vi "All Values.vi"(8 "error in (no error)":errorcluster, 11 "Group in":refnum<class "Group DBL.lvclass">) -> (0 "error out":errorcluster, 1 "Timestamp":dbl[](array[numeric]), 2 "Scaled":dbl[](array[numeric]), 3 "Group out":refnum<class "Group DBL.lvclass">, 4 "Raw":dbl[](array[numeric]))   [LabVIEW 2020, in "Vecto.lvlib" / "Group DBL.lvclass"]
uses:
  Group DBL.lvclass
  Group DBL.lvclass/Group DBL.ctl
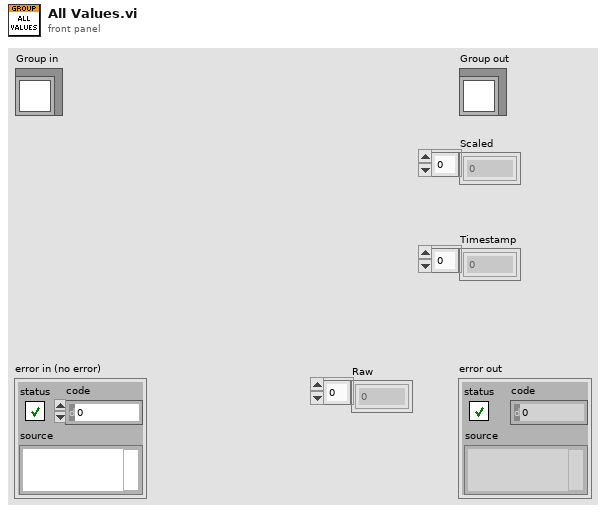
[diagram p1: front panel]
types:
  T1 = typedef "Vecto.lvlib/Group.lvclass/Ref.ctl" = cluster{"Scaled":dbl[], "Timestamp":dbl[], "Raw":dbl[]}
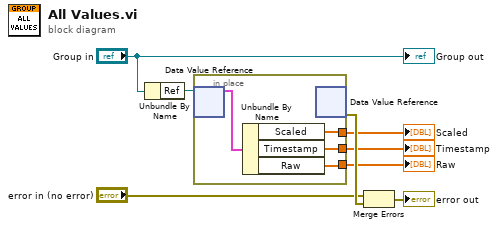
[diagram p0: block diagram]
diagram:
  n1 = Unbundle By Name("Group in") -> ("Ref"=w6:refnum<data-value>)
  n2 = in-place {
    in-place-border: [w12] -> w3
    in-place-border: [w11] -> w2
    in-place-border: [w10] -> w1
    n3 = in-place-dvr #1(w6) -> (w9:T1)  [unwired: 1 out]
    n4 = Unbundle By Name(w9) -> ("Scaled"=w12:dbl[], "Timestamp"=w11:dbl[], "Raw"=w10:dbl[])
    n5 = in-place-dvr #1() -> (w8:errorcluster)  [unwired: 1 in, 1 out]
  }
  "Scaled" <- w3
  "Timestamp" <- w2
  "Raw" <- w1
  n6 = Merge Errors("error in (no error)", w8) -> (→"error out":errorcluster)
  "Group out" <- "Group in"
